vi "Check Running State.vi"(8 "error in (no error)":errorcluster, 11 "Panel State Data In":T1) -> (0 "error out":errorcluster, 2 "Is Done?":bool, 3 "Panel State Data Out":T1)   [LabVIEW 2025]
uses:
  Typedef/Test Panel State Data.ctl
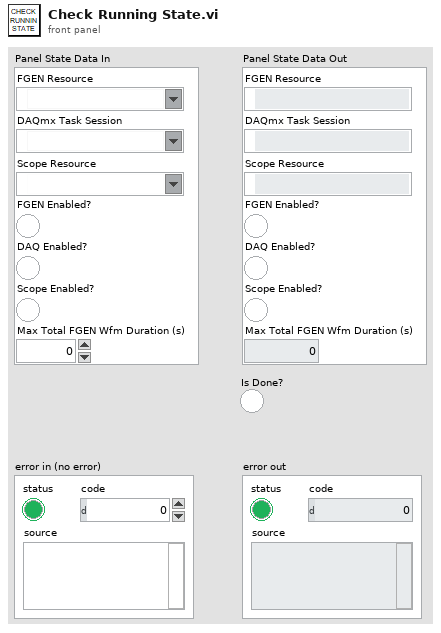
[diagram p1: front panel]
types:
  T1 = typedef "Test Panel State Data.ctl" = cluster{"FGEN Resource":refnum<k15>, "DAQmx Task Session":refnum<k21>, "Scope Resource":refnum<k15>, "FGEN Enabled?":bool, "DAQ Enabled?":bool, "Scope Enabled?":bool, "Max Total FGEN Wfm Duration (s)":dbl}
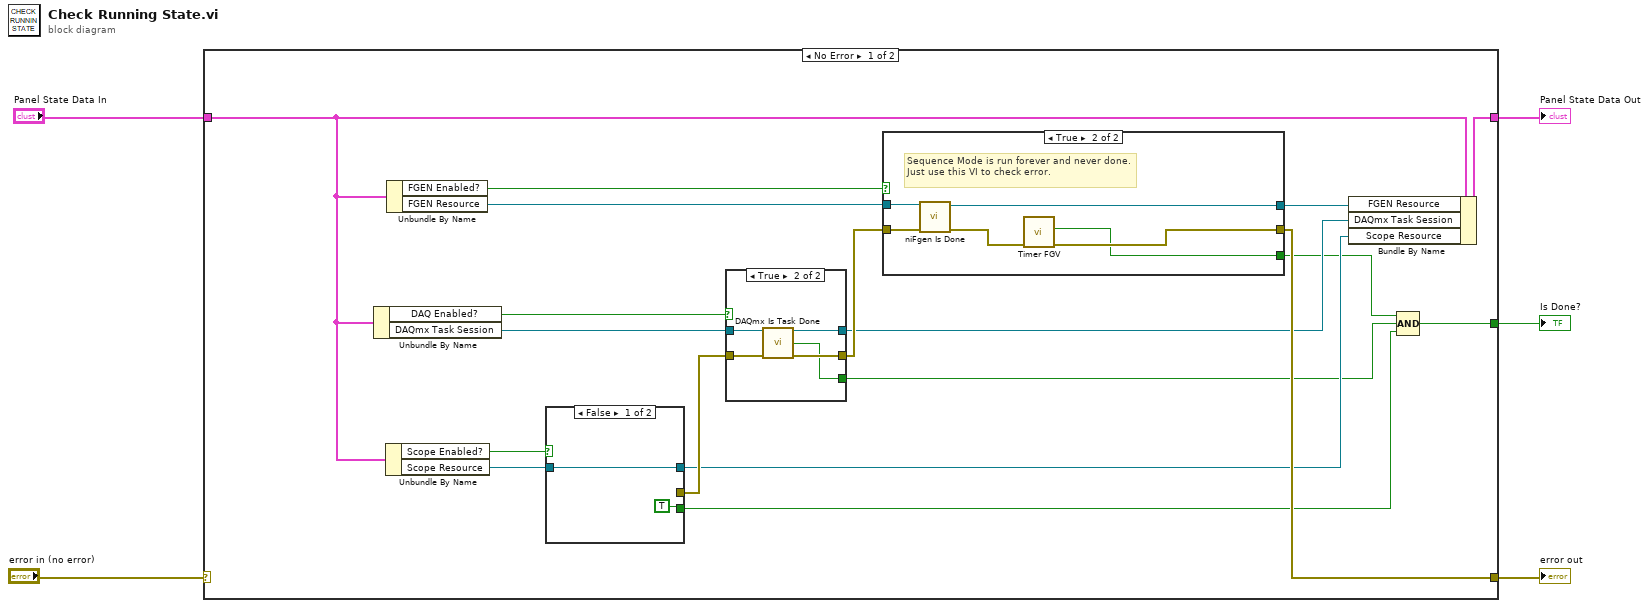
[diagram p0: block diagram]
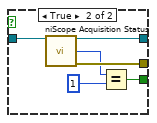
[diagram p2: hidden frame]
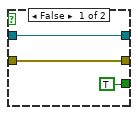
[diagram p3: hidden frame]
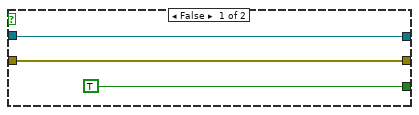
[diagram p4: hidden frame]
diagram:
  n1 = case shown="No Error" "error in (no error)" {
    selector: "error in (no error)" -> [_ w50]
    tunnel: "Panel State Data In" -> [w17 w49]
    tunnel: [w14 w50] -> w3
    tunnel: [w13 w49] -> w4
    tunnel: [w6 _] -> w1
    frame No Error {
      n2 = Unbundle By Name(w17) -> ("DAQ Enabled?"=w20:bool, "DAQmx Task Session"=w21:refnum<k21>)
      n3 = Unbundle By Name(w17) -> ("Scope Enabled?"=w19:bool, "Scope Resource"=w18:refnum<k15>)
      n4 = Unbundle By Name(w17) -> ("FGEN Enabled?"=w23:bool, "FGEN Resource"=w22:refnum<k15>)
      n5 = case shown="False" w19 {
        tunnel: w18 -> [w25 w30]
        tunnel: [_ w31] -> w16
        tunnel: [w25 w29] -> w10
        tunnel: [TRUE w26] -> w7
        frame False {
        }
        frame True {
          n6 = call <instrlib>:"niScope Acquisition Status.vi"("instrument handle"=w30) -> ("instrument handle out"=w29:refnum<k15>, "acquisition status"=w27:i32, "error out"=w31:errorcluster)  [unwired: 12 in]
          n7 = Equal?(x=w27, y=1 ("acquisition status")) -> (x = y?=w26:bool)
        }
      }
      n8 = case shown="True" w20 {
        tunnel: w21 -> [w33 w39]
        tunnel: [w34 w38] -> w15
        tunnel: w16 -> [w34 w37]
        tunnel: [w33 w36] -> w11
        tunnel: [TRUE ("task done?") w35] -> w8
        frame False {
        }
        frame True {
          n9 = call <vilib>:"DAQmx Is Task Done.vi"("task/channels in"=w39, "error in"=w37) -> ("task out"=w36:refnum<k21>, "task done?"=w35:bool, "error out"=w38:errorcluster)  [unwired: 11 in]
        }
      }
      n10 = case shown="True" w23 {
        tunnel: w22 -> [w41 w48]
        tunnel: [w42 w44] -> w14
        tunnel: w15 -> [w42 w46]
        tunnel: [w41 w45] -> w12
        tunnel: [TRUE ("Done") w43] -> w9
        frame False {
        }
        frame True {
          # "Sequence Mode is run forever and never done. Just use this VI to check error."
          n11 = call <instrlib>:"niFgen Is Done.vi"("error in (no error)"=w46, "Instrument Handle"=w48) -> ("error out"=w47:errorcluster, "Instrument Handle Out"=w45:refnum<k15>)  [unwired: 7 in, 1 out]
          n12 = call "Timer FGV.vi"("error in (no error)"=w47) -> ("error out"=w44:errorcluster, "Time Elapsed?"=w43:bool)  [unwired: 7 in, 2 out]
        }
      }
      n13 = Bundle By Name(cluster=w17, "FGEN Resource"=w12, "DAQmx Task Session"=w11, "Scope Resource"=w10) -> (w13:T1)
      n14 = Compound Arithmetic op=AND(w9, w8, w7) -> (w6:bool)
    }
    frame Error {
    }
  }
  "error out" <- w3
  "Panel State Data Out" <- w4
  "Is Done?" <- w1
